vi "Zero_Turret_Spin.vi"(1 "Zero_Turret_Spin":bool, 3 "Turret Motor Ref":T1, 4 "Pulse Width Position":i32) -> ()   [LabVIEW 2020]
uses:
  <vilib>/Rock Robotics/WPI/MotorControl/WPI_MotorControlDeviceRef.ctl
  <vilib>/Rock Robotics/WPI/MotorControl/WPI_MotorControlType.ctl
  <vilib>/Rock Robotics/SystemInterfaces/DIO/FPGA_DIOPWMChannel.ctl
  <vilib>/Rock Robotics/WPI/PWM/WPI_PWMDeadband.ctl
  <vilib>/Rock Robotics/SystemInterfaces/DIO/FPGA_DIOChannel.ctl
  Globals/Sensor_Values.vi
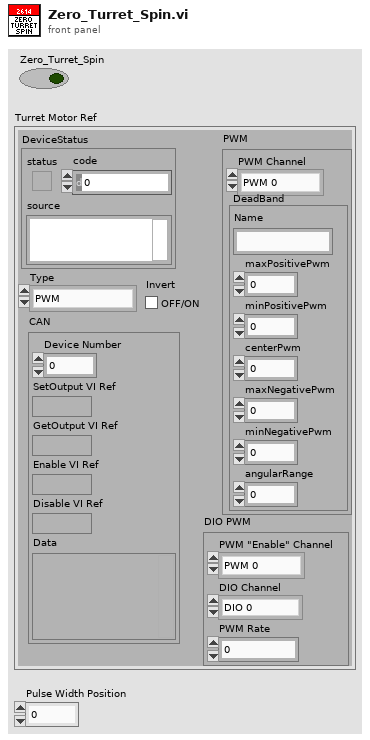
[diagram p1: front panel]
types:
  T1 = typedef "WPI_MotorControlDeviceRef.ctl" = cluster{"DeviceStatus":errorcluster, "Type":T2, "PWM":cluster{"PWM Channel":T3, "DeadBand":T4}, "CAN":cluster{"Device Number":u8, "SetOutput VI Ref":variant, "GetOutput VI Ref":variant, "Enable VI Ref":variant, "Disable VI Ref":variant, "Data":variant}, "Invert":bool, "DIO PWM":cluster{"PWM \"Enable\" Channel":T3, "DIOChannel":T5, "PWM Rate":dbl}}
  T2 = typedef "WPI_MotorControlType.ctl" = enum16{"PWM", "CAN", "DIO PWM"}
  T3 = typedef "FPGA_DIOPWMChannel.ctl" = enum8{"PWM 0", "PWM 1", "PWM 2", "PWM 3", "PWM 4", "PWM 5", "PWM 6", "PWM 7", "PWM 8", "PWM 9", "PWM MXP 0", "PWM MXP 1", "PWM MXP 2", "PWM MXP 3", "PWM MXP 4", "PWM MXP 5", "PWM MXP 6", "PWM MXP 7", "PWM MXP 8", "PWM MXP 9", "Invalid"}
  T4 = typedef "WPI_PWMDeadband.ctl" = cluster{"Name":string, "maxPositivePwm":i32, "minPositivePwm":i32, "centerPwm":i32, "maxNegativePwm":i32, "minNegativePwm":i32, "angularRange":u16}
  T5 = typedef "FPGA_DIOChannel.ctl" = enum8{"DIO 0", "DIO 1", "DIO 2", "DIO 3", "DIO 4", "DIO 5", "DIO 6", "DIO 7", "DIO 8", "DIO 9", "DIO MXP 0", "DIO MXP 1", "DIO MXP 2", "DIO MXP 3", "DIO MXP 4", "DIO MXP 5", "DIO MXP 6", "DIO MXP 7", "DIO MXP 8", "DIO MXP 9", "DIO MXP 10", "DIO MXP 11", "DIO MXP 12", "DIO MXP 13", "DIO MXP 14", "DIO MXP 15", "SPI Port CS1", "SPI Port CS2", "SPI Port CS3", "SPI Port MISO", "SPI Port MOSI", "Invalid"}
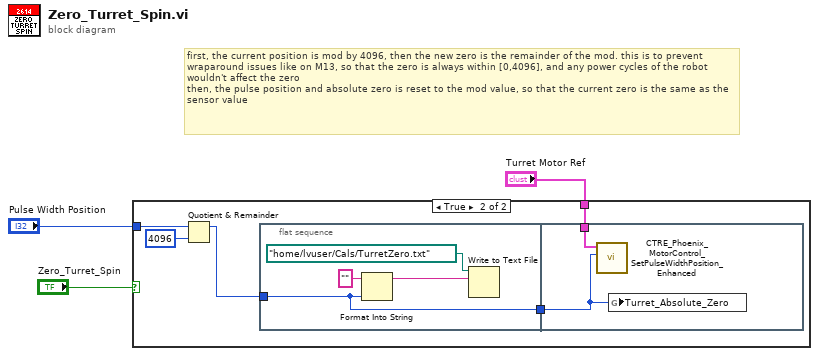
[diagram p0: block diagram]
diagram:
  # "first, the current position is mod by 4096, then the new zero is the remainder of the mod. this is to prevent wraparound issues like on M13, so that the zero is always within [0,4096], and any power cycles of the robot wouldn't affect the zero\nthen, the pulse position and absolute zero is reset to the mod value, so that the current zero is the same as the sensor value"
  n1 = case shown="True" "Zero_Turret_Spin" {
    tunnel: "Pulse Width Position" -> [_ w8]
    tunnel: "Turret Motor Ref" -> [_ w4]
    frame False {
    }
    frame True {
      n2 = Quotient & Remainder(x=w8, y=4096) -> (x-y*floor(x/y)=w6:i32)  [unwired: 1 out]
      n3 = flat-sequence {
        tunnel: w6 -> [w9]
        tunnel: [w9] -> w5
        tunnel: w5 -> [w13]
        tunnel: w4 -> [w14]
        frame #0 {
          n4 = Format Into String(initial string="", w9) -> (resulting string=w10:string)  [unwired: 2 in, 1 out]
          n5 = Write to Text File(file (use dialog)=path "/home/lvuser/Cals/TurretZero.txt", text=w10) -> ()  [unwired: 2 in, 3 out]
        }
        frame #1 {
          n6 = call <vilib>:"CTRE_Phoenix_MotorControl_SetPulseWidthPosition_Enhanced.vi"("New Position"=w13, "PhoenixMotorControlDevRef"=w14) -> ()  [unwired: 8 in, 2 out]
          n7 = global write "Sensor_Values.vi" "Turret_Absolute_Zero"(w13) -> ()
        }
      }
    }
  }
